vi "CurrentANDvoltage_readings.vi"() -> ()   [LabVIEW 2017]
uses:
  <vilib>/Analysis/baseanly.llb/Mean (DBL).vi
  <instrlib>/Keithley 6517/Keithley 6517.lvlib
  <vilib>/Analysis/NI_AALBase.lvlib
panel:
  out "Array 3":string[](array[string])
  out "appended array":ext[](array[numeric])
  out "Resistance MEAN 2":dbl=7279.3150000000005
  out "ERROR 2":dbl=7279.3150000000005
  out "Current MEAN 2":dbl=7279.3150000000005
  out "ERROR":dbl=7279.3150000000005
  out "Voltage MEAN":dbl=7279.3150000000005
  out "Array 2":dbl[](array[numeric])
  out "XY Graph":cluster{dbl[], ext[]}(graph)
  in  "V-source Amplitude":dbl format="%.6e"
  out "Array":dbl[](array[numeric])
  in  "?":dbl
  in  "milliseconds to wait":u32
  in  "VISA resource name 2":refnum<visa-resource-name>
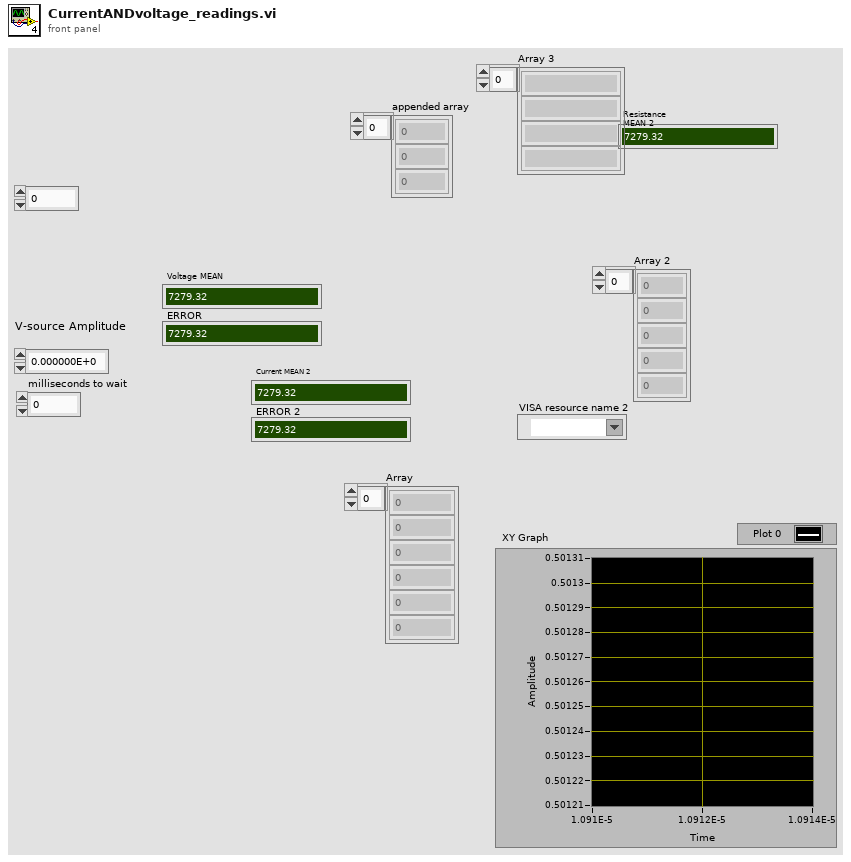
[diagram p1: front panel]
types:
  T1 = cluster{"Measurement":dbl, "Units":string, "Time Stamp and Date":string, "Reading #":dbl, "Channel #":dbl}
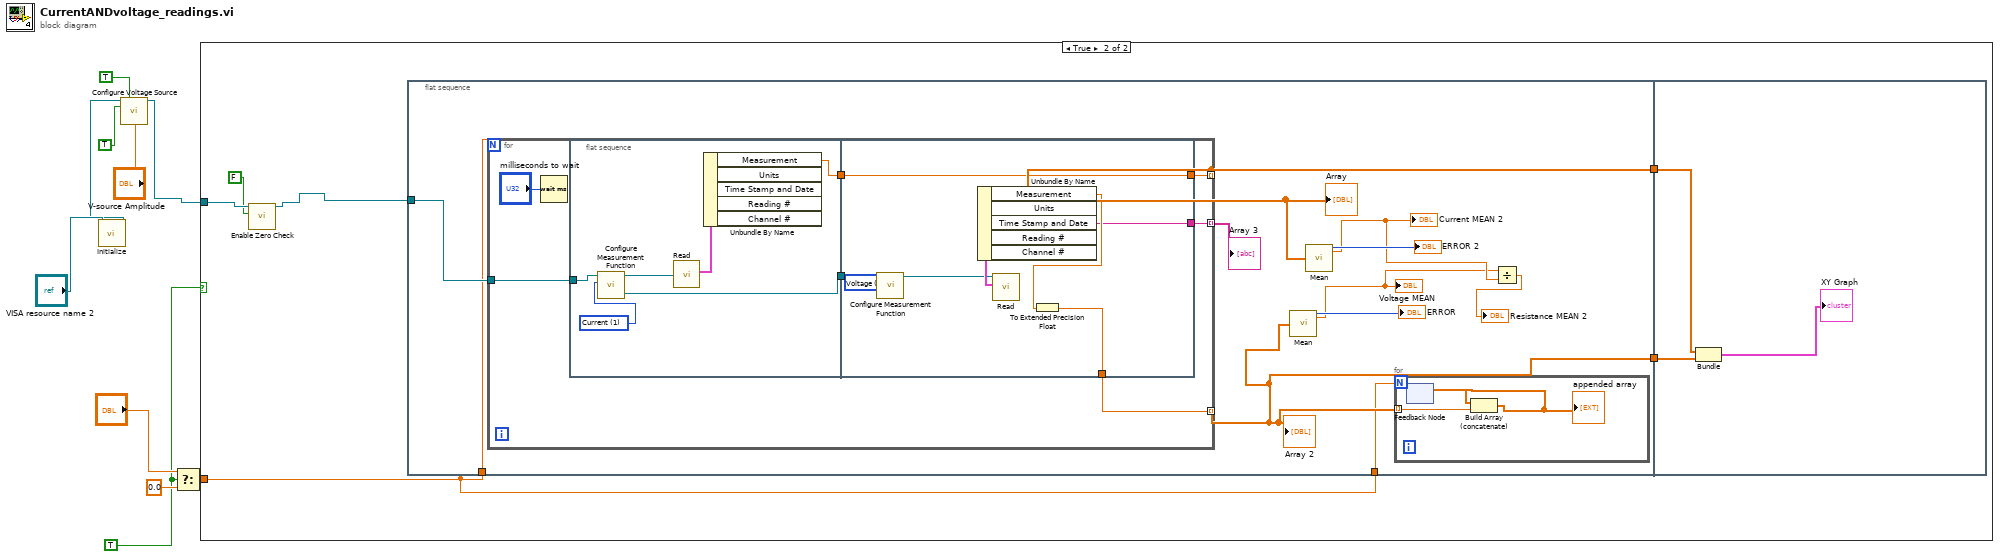
[diagram p0: block diagram]
diagram:
  w6 = TRUE
  n1 = call <instrlib>:"Initialize.vi"("VISA resource name"="VISA resource name 2") -> ("VISA resource name out"=w5:refnum<visa-resource-name>)  [unwired: 9 in, 1 out]
  n2 = call <instrlib>:"Configure Voltage Source.vi"("VISA resource name"=w5, "Enable LO Connection (F: Disable)"=TRUE, "Enable V-source (F: Disable)"=TRUE, "V-source Amplitude (0.000000E+0)"="V-source Amplitude") -> ("VISA resource name out"=w4:refnum<visa-resource-name>)  [unwired: 10 in, 1 out]
  n3 = Select(t="?", s=w6, f=0.0) -> (s? t:f=w8:dbl)
  n4 = case shown="True" w6 {
    tunnel: w4 -> [_ w16]
    tunnel: w8 -> [_ w11]
    frame False {
    }
    frame True {
      n5 = call <instrlib>:"Enable Zero Check.vi"("Enable Zero Check (T: Enable)"=FALSE, "VISA resource name"=w16) -> ("VISA resource name out"=w15:refnum<visa-resource-name>)  [unwired: 8 in, 1 out]
      n6 = flat-sequence {
        tunnel: w15 -> [w27]
        tunnel: w11 -> [w26]
        tunnel: [w23] -> w13
        tunnel: [w19] -> w12
        tunnel: w11 -> [w18]
        tunnel: w13 -> [w53]
        tunnel: w12 -> [w52]
        frame #0 {
          n7 = for {
            N: w26 -> [_]
            tunnel: w27 -> [w35]
            tunnel: [w36] -> w23 mode=indexing
            tunnel: [w32] -> w19 mode=indexing
            tunnel: [w31] -> w17 mode=indexing
            n8 = Wait (ms)(milliseconds to wait="milliseconds to wait") -> ()  [unwired: 1 out]
            n9 = flat-sequence {
              tunnel: w35 -> [w40]
              tunnel: [w41] -> w34
              tunnel: [w39] -> w33
              tunnel: [w50] -> w36
              tunnel: w34 -> [w50]
              tunnel: w33 -> [w47]
              tunnel: [w44] -> w32
              tunnel: [w43] -> w31
              frame #0 {
                w38 = 1 items=["Voltage", "Current", "Resistance", "Charge"] ("Measurement Function (0: Voltage)")
                n10 = call <instrlib>:"Configure Measurement Function.vi"("Measurement Function (0: Voltage)"=w38, "VISA resource name"=w40) -> ("VISA resource name out"=w39:refnum<visa-resource-name>)  [unwired: 8 in, 1 out]
                n11 = call <instrlib>:"Read.vi"("VISA resource name"=w39) -> ("Measurement"=w42:T1)  [unwired: 8 in, 2 out]
                n12 = Unbundle By Name(w42) -> ("Measurement"=w41:dbl)  [unwired: 4 out]
              }
              frame #1 {
                w46 = 0 items=["Voltage", "Current", "Resistance", "Charge"] ("Measurement Function (0: Voltage)")
                n13 = call <instrlib>:"Configure Measurement Function.vi"("Measurement Function (0: Voltage)"=w46, "VISA resource name"=w47) -> ("VISA resource name out"=w48:refnum<visa-resource-name>)  [unwired: 8 in, 1 out]
                n14 = call <instrlib>:"Read.vi"("VISA resource name"=w48) -> ("Measurement"=w49:T1)  [unwired: 8 in, 2 out]
                n15 = Unbundle By Name(w49) -> ("Measurement"=w45:dbl, "Time Stamp and Date"=w43:string)  [unwired: 3 out]
                n16 = To Extended Precision Float(1:w45) -> (0:w44:ext)
              }
            }
          }
          "Array" <- w23
          "Array 2" <- w19
          "Array 3" <- w17
          n17 = call-poly <vilib>:"Mean.vi"("X"=w19) -> ("mean"=w21:dbl, "error"=→"ERROR":i32)
          "Voltage MEAN" <- w21
          n18 = call-poly <vilib>:"Mean.vi"("X"=w23) -> ("mean"=w22:dbl, "error"=→"ERROR 2":i32)
          "Current MEAN 2" <- w22
          n19 = for {
            N: w18 -> [_]
            tunnel: w19 -> [w30] mode=indexing
            n20 = feedback #1() -> (w29:ext[])  [unwired: 1 in]
            n21 = Build Array (concatenate)(w29, w30) -> (w28:ext[])
            "appended array" <- w28
            n22 = feedback-in #1(w28) -> ()
          }
          n23 = Divide(x=w21, y=w22) -> (x/y=→"Resistance MEAN 2":dbl)
        }
        frame #1 {
          n24 = Bundle(w53, w52) -> (→"XY Graph":cluster{dbl[], ext[]})  [unwired: 1 in]
        }
      }
    }
  }
